vi "UpdateLEDsOnChange.vi"(6 "LED1":bool, 7 "LED0":bool, 8 "error in":errorcluster, 9 "LED1 current":string(combo)="0", 10 "LED0 current":string(combo)="0", 11 "VISA resource name in":refnum<visa-resource-name>) -> (0 "error out":errorcluster, 3 "VISA resource name out":refnum<visa-resource-name>)   [LabVIEW 2011]
panel:
  out "Boolean":bool=TRUE
  out "data to write":string
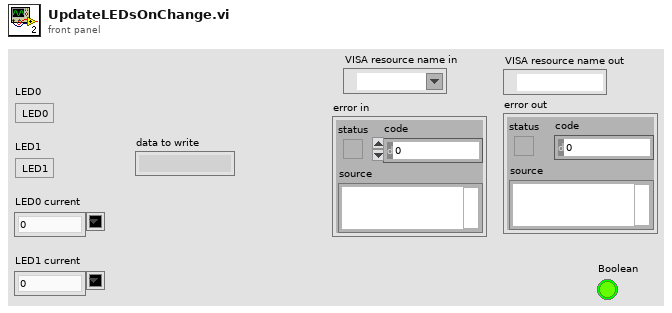
[diagram p1: front panel]
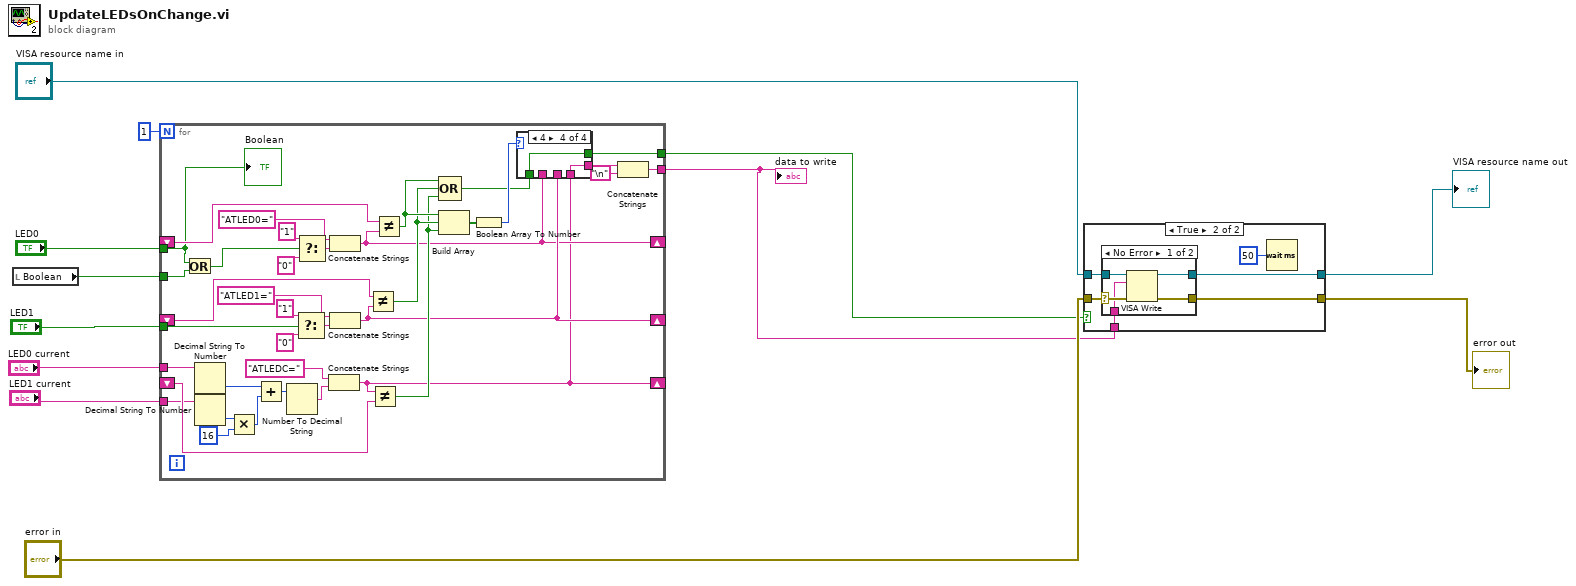
[diagram p0: block diagram]
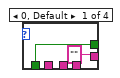
[diagram p4: hidden frame]
diagram:
  n1 = local read "Boolean"() -> (w1:bool)
  n2 = for {
    N: 1 -> [_]
    shift-right: [w21] -> _
    shift-left: _ -> [w26]
    shift-right: [w25] -> _
    shift-left: _ -> [w22]
    shift-right: [w24] -> _
    shift-left: _ -> [w23]
    tunnel: [w20] -> w2
    tunnel: [w19] -> w3
    tunnel: "LED0 current" -> [w18]
    tunnel: "LED1 current" -> [w17]
    tunnel: "LED0" -> [w13]
    tunnel: "LED1" -> [w16]
    tunnel: w1 -> [w15]
    n3 = Or(x=w13, y=w15) -> (x .or. y?=w14:bool)
    n4 = Decimal String To Number(string=w18) -> (number=w37:i32)  [unwired: 2 in, 1 out]
    n5 = Decimal String To Number(string=w17) -> (number=w40:i32)  [unwired: 2 in, 1 out]
    n6 = Multiply(x=w40, y=16) -> (x*y=w38:i32)
    n7 = Add(x=w37, y=w38) -> (x+y=w36:i32)
    n8 = Number To Decimal String(number=w36) -> (decimal integer string=w35:string)  [unwired: 1 in]
    n9 = Select(t="1", s=w16, f="0") -> (s? t:f=w43:string)
    n10 = Select(t="1", s=w14, f="0") -> (s? t:f=w45:string)
    n11 = Concatenate Strings("ATLEDC=", w35) -> (w21:string)
    n12 = Concatenate Strings("ATLED0=", w45) -> (w24:string)
    n13 = Concatenate Strings("ATLED1=", w43) -> (w25:string)
    n14 = Not Equal?(x=w22, y=w25) -> (x != y?=w29:bool)
    n15 = Not Equal?(x=w21, y=w26) -> (x != y?=w28:bool)
    n16 = Not Equal?(x=w23, y=w24) -> (x != y?=w30:bool)
    n17 = Compound Arithmetic op=OR(w30, w29, w28) -> (w27:bool)
    n18 = Build Array(w30, w29, w28) -> (w41:bool[])
    n19 = Boolean Array To Number(Boolean array=w41) -> (number=w33:u32)
    n20 = case shown="4" w33 {
      tunnel: ["" w53 w55 w57] -> w31
      tunnel: w24 -> [_ w53 _ _]
      tunnel: w25 -> [_ _ w55 _]
      tunnel: w21 -> [_ _ _ w57]
      tunnel: [w50 w52 w54 w56] -> w19
      tunnel: w27 -> [w50 w52 w54 w56]
      frame 0, Default {
      }
      frame 1 {
      }
      frame 2 {
      }
      frame 4 {
      }
    }
    n21 = Concatenate Strings(w31, "\n") -> (w20:string)
    "Boolean" <- w13
  }
  "data to write" <- w2
  n22 = case shown="True" w3 {
    tunnel: [w59 w65] -> w6
    tunnel: [w58 w64] -> w7
    tunnel: "VISA resource name in" -> [w59 w63]
    tunnel: "error in" -> [w58 w62]
    tunnel: w2 -> [_ w61]
    frame False {
    }
    frame True {
      n23 = case shown="No Error" w62 {
        selector: w62 -> [w67 w72]
        tunnel: [w70 w71] -> w65
        tunnel: [w69 w72] -> w64
        tunnel: w63 -> [w68 w71]
        tunnel: w61 -> [w66 _]
        frame No Error {
          n24 = VISA Write(VISA resource name=w68, write buffer=w66, error in (no error)=w67) -> (VISA resource name out=w70:refnum<visa-resource-name>, error out=w69:errorcluster)  [unwired: 1 out]
        }
        frame Error {
        }
      }
      n25 = Wait (ms)(milliseconds to wait=u32 50) -> ()  [unwired: 1 out]
    }
  }
  "VISA resource name out" <- w6
  "error out" <- w7
